vi "ADI_IMU_ADIS16470_OffsetComp.vi"(6 "error in":errorcluster, 8 "Bytes per Sample":u32, 9 "n Samples":u32=1000) -> (0 "error out":errorcluster, 1 "Sensor Ready?":bool, 2 "Offsets":dbl[](array[numeric]), 3 "Timestamp":u32)   [LabVIEW 2018, in "ADIS16470_IMU.lvlib"]
uses:
  ADIS16470_IMU.lvlib
  <vilib>/Rock Robotics/SystemInterfaces/DIO/FPGA_DIOChannel.ctl
  <vilib>/Analysis/baseanly.llb/Mean (DBL).vi
  <vilib>/Analysis/NI_AALBase.lvlib
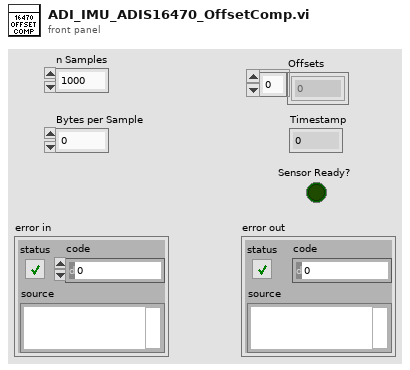
[diagram p1: front panel]
types:
  T1 = typedef "FPGA_DIOChannel.ctl" = enum8{"DIO 0", "DIO 1", "DIO 2", "DIO 3", "DIO 4", "DIO 5", "DIO 6", "DIO 7", "DIO 8", "DIO 9", "DIO MXP 0", "DIO MXP 1", "DIO MXP 2", "DIO MXP 3", "DIO MXP 4", "DIO MXP 5", "DIO MXP 6", "DIO MXP 7", "DIO MXP 8", "DIO MXP 9", "DIO MXP 10", "DIO MXP 11", "DIO MXP 12", "DIO MXP 13", "DIO MXP 14", "DIO MXP 15", "SPI Port CS1", "SPI Port CS2", "SPI Port CS3", "SPI Port MISO", "SPI Port MOSI", "Invalid"}
  T2 = typedef "WPI_DigitalOutputDevRef.ctl" = cluster{"DIO Channel":T1, "DevStatus":errorcluster}
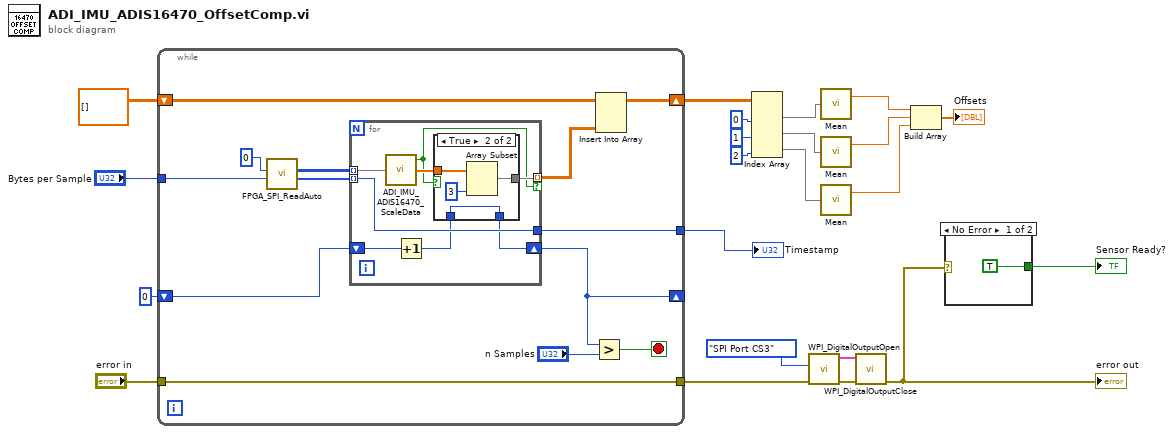
[diagram p0: block diagram]
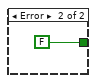
[diagram p2: hidden frame]
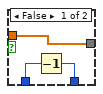
[diagram p3: hidden frame]
diagram:
  n1 = while {
    shift-right: [w31] -> w11
    shift-left: dbl[][] [] -> [w30]
    shift-right: [w25] -> _
    shift-left: u32 0 -> [w26]
    tunnel: "Bytes per Sample" -> [w27]
    tunnel: [w24] -> w8
    tunnel: [w23] -> w4
    tunnel: "error in" -> [w23]
    stop <- w28 stop-if-true
    n2 = call <vilib>:"FPGA_SPI_ReadAuto.vi"("Bytes per Sample"=w27, "Samples to Read"=u32 0) -> ("Timestamps"=w33:u32[], "Data"=w34:u8[][])  [unwired: 7 in, 1 out]
    n3 = for {
      tunnel: w34 -> [w43] mode=indexing
      tunnel: [w41] -> w32 mode=indexing if=w36
      tunnel: w33 -> [w40] mode=indexing
      tunnel: [w40] -> w24
      shift-right: [w37] -> w25
      shift-left: w26 -> [w39]
      n4 = call "ADI_IMU_ADIS16470_ScaleData.vi"("Received Data"=w43) -> ("Data Array"=w42:dbl[], "Data Good?"=w36:bool)  [unwired: 2 in, 1 out]
      n5 = Increment(x=w39) -> (x+1=w38:u32)
      n6 = case shown="True" w36 {
        tunnel: w42 -> [w46 w50]
        tunnel: [w46 w48] -> w41
        tunnel: w38 -> [w45 w47]
        tunnel: [w44 w47] -> w37
        frame False {
          n7 = Decrement(x=w45) -> (x-1=w44:u32)
        }
        frame True {
          n8 = Array Subset(array=w50, length=3) -> (w48:dbl[])  [unwired: 1 in]
        }
      }
    }
    n9 = Greater?(x=w25, y="n Samples") -> (0:w28:bool)
    n10 = Insert Into Array(array=w30, new element=w32) -> (w31:dbl[][])  [unwired: 2 in]
  }
  "Timestamp" <- w8
  n11 = Index Array(array=w11, index (col) #1=0 ("disabled index (col)"), index (col) #2=1 ("index (col)"), index (col) #3=2 ("index (col)")) -> (element #1=w17:dbl[], element #2=w16:dbl[], element #3=w15:dbl[])  [unwired: 3 in]
  n12 = call <vilib>:"WPI_DigitalOutputOpen.vi"("error in (no error)"=w4, "DIO Channel"=FPGA_DIOChannel."SPI Port CS3") -> ("error out"=w6:errorcluster, "DigitalOutputDevRef"=w7:T2)  [unwired: 8 in]
  n13 = call-poly <vilib>:"Mean.vi"("X"=w17) -> ("mean"=w14:dbl)  [unwired: 1 out]
  n14 = call-poly <vilib>:"Mean.vi"("X"=w16) -> ("mean"=w13:dbl)  [unwired: 1 out]
  n15 = call-poly <vilib>:"Mean.vi"("X"=w15) -> ("mean"=w12:dbl)  [unwired: 1 out]
  n16 = call <vilib>:"WPI_DigitalOutputClose.vi"("error in (no error)"=w6, "DigitalOutputDevRef"=w7) -> ("error out"=w2:errorcluster)  [unwired: 9 in]
  "error out" <- w2
  n17 = Build Array(w14, w13, w12) -> (→"Offsets":dbl[])
  n18 = case shown="No Error" w2 {
    tunnel: [TRUE FALSE] -> w1
    frame No Error {
    }
    frame Error {
    }
  }
  "Sensor Ready?" <- w1
